vi "Get NET Object--Accessor.vi"(8 "error in (no error)":errorcluster, 11 "Watlow F4T in":refnum<class "Watlow F4T.lvclass">) -> (0 "error out":errorcluster, 2 ".NET Object":refnum<k24>, 3 "Watlow F4T out":refnum<class "Watlow F4T.lvclass">)   [LabVIEW 2024, in "Watlow F4T.lvclass"]
uses:
  Watlow F4T.lvclass
  <instrlib>/Watlow Std Bus/Public/Watbus.dll
  Watlow F4T.lvclass/Watlow F4T.ctl
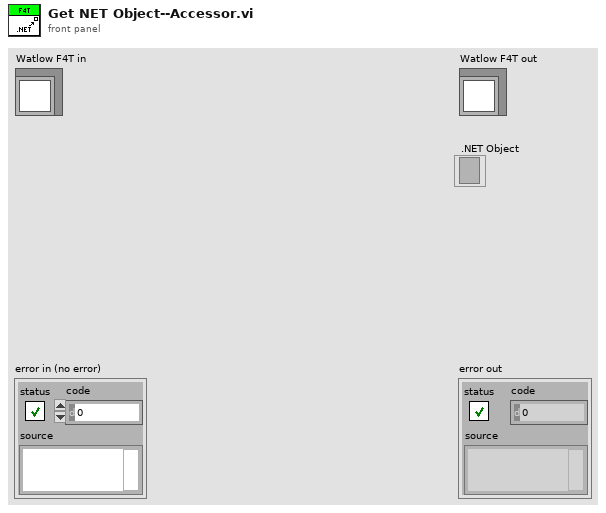
[diagram p1: front panel]
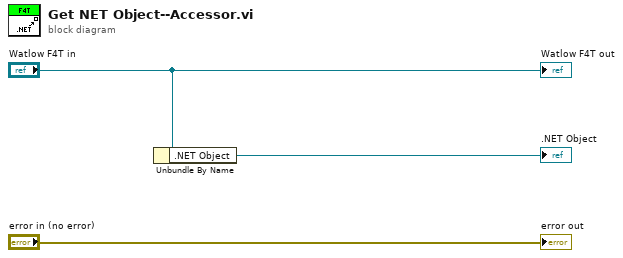
[diagram p0: block diagram]
diagram:
  n1 = Unbundle By Name("Watlow F4T in") -> (".NET Object"=→".NET Object":refnum<k24>)
  "error out" <- "error in (no error)"
  "Watlow F4T out" <- "Watlow F4T in"
